vi "VI Tree.vi"   [LabVIEW 2012, in "Lake Shore Cryotronics 218.lvlib"]
doc: "This is the instrument driver for the LakeShore Cryotronics Model 218 Temperature Monitor. The VI Tree displays all the user-callable VIs of the instrument driver in an organized table.\n\nThis Instrument Driver's Revision number is \"REV 1.0, 01/1999, LV 5.0\" and is compatible with Instrument Firmware Revision: \"M218F 07/15/98\" and later.\n\nLakeShore Cryotronics Model 218 Temperature Monitor\nCreated By: Rob Welsh\nRelease Date: January 1999\nOriginally Developed in LabVIEW Version: 5.0\n\nModification History: \n\nNone"
uses:
  <instrlib>/Lake Shore Cryotronics 218/Lake Shore Cryotronics 218.lvlib
panel:
  # "© 2005 National Instruments.  ALL RIGHTS RESERVED."
  # "SEE DIAGRAM\nFOR VI TREE."
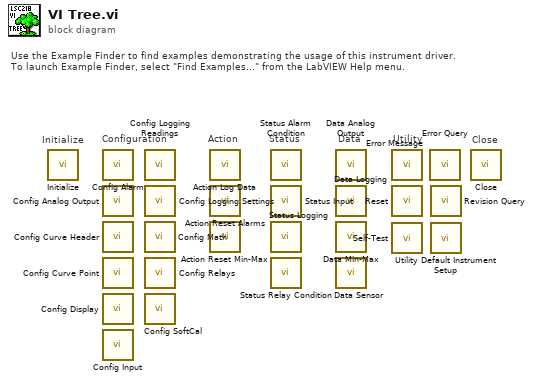
[diagram p0: block diagram]
diagram:
  # "Status"
  # "Initialize"
  # "Close"
  # "Action"
  # "Data"
  # "Utility"
  # "Configuration"
  # "Use the Example Finder to find examples demonstrating the usage of this instrument driver.\nTo launch Example Finder, select \"Find Examples...\" from the LabVIEW Help menu."
  n1 = call <instrlib>:"Initialize.vi"() -> ()  [unwired: 14 in, 2 out]
  n2 = call <instrlib>:"Config Alarm.vi"() -> ()  [unwired: 14 in, 2 out]
  n3 = call <instrlib>:"Config Analog Output.vi"() -> ()  [unwired: 14 in, 2 out]
  n4 = call <instrlib>:"Config Curve Header.vi"() -> ()  [unwired: 14 in, 2 out]
  n5 = call <instrlib>:"Config Curve Point.vi"() -> ()  [unwired: 14 in, 2 out]
  n6 = call <instrlib>:"Config Display.vi"() -> ()  [unwired: 14 in, 2 out]
  n7 = call <instrlib>:"Config Input.vi"() -> ()  [unwired: 14 in, 2 out]
  n8 = call <instrlib>:"Config Logging Readings.vi"() -> ()  [unwired: 14 in, 2 out]
  n9 = call <instrlib>:"Config Logging Settings.vi"() -> ()  [unwired: 14 in, 2 out]
  n10 = call <instrlib>:"Config Math.vi"() -> ()  [unwired: 14 in, 2 out]
  n11 = call <instrlib>:"Config Relays.vi"() -> ()  [unwired: 14 in, 2 out]
  n12 = call <instrlib>:"Config SoftCal.vi"() -> ()  [unwired: 14 in, 2 out]
  n13 = call <instrlib>:"Action Log Data.vi"() -> ()  [unwired: 14 in, 2 out]
  n14 = call <instrlib>:"Action Reset Alarms.vi"() -> ()  [unwired: 14 in, 2 out]
  n15 = call <instrlib>:"Action Reset Min-Max.vi"() -> ()  [unwired: 14 in, 2 out]
  n16 = call <instrlib>:"Status Alarm Condition.vi"() -> ()  [unwired: 11 in, 5 out]
  n17 = call <instrlib>:"Status Input.vi"() -> ()  [unwired: 11 in, 5 out]
  n18 = call <instrlib>:"Status Logging.vi"() -> ()  [unwired: 12 in, 4 out]
  n19 = call <instrlib>:"Status Relay Condition.vi"() -> ()  [unwired: 13 in, 3 out]
  n20 = call <instrlib>:"Data Analog Output.vi"() -> ()  [unwired: 13 in, 3 out]
  n21 = call <instrlib>:"Data Logging.vi"() -> ()  [unwired: 9 in, 7 out]
  n22 = call <instrlib>:"Data Min-Max.vi"() -> ()  [unwired: 12 in, 4 out]
  n23 = call <instrlib>:"Data Sensor.vi"() -> ()  [unwired: 6 in, 10 out]
  n24 = call <instrlib>:"Error Message.vi"() -> ()  [unwired: 11 in, 5 out]
  n25 = call <instrlib>:"Reset.vi"() -> ()  [unwired: 14 in, 2 out]
  n26 = call <instrlib>:"Self-Test.vi"() -> ()  [unwired: 12 in, 4 out]
  n27 = call <instrlib>:"Error Query.vi"() -> ()  [unwired: 12 in, 4 out]
  n28 = call <instrlib>:"Revision Query.vi"() -> ()  [unwired: 10 in, 6 out]
  n29 = call <instrlib>:"Utility Default Instrument Setup.vi"() -> ()  [unwired: 14 in, 2 out]
  n30 = call <instrlib>:"Close.vi"() -> ()  [unwired: 15 in, 1 out]
